vi "COD内部交互全局.vi"() -> ()   [LabVIEW 2016, in "斯坦道CODMn.lvlib"]
panel:
  in  "PID参数":cluster{"P":dbl, "I":dbl, "D":dbl}
  out "F0-F5":u16[](array[numeric])
  in  "更换泵管":bool
  out "采水泵参数":i32[](array[numeric])
  in  "泵校准参数":T1
  in  "保存参数":dbl[](array[numeric])
  in  "选项卡控件":enum32{"滴定曲线", "温度曲线"}(tab)
  out "ORP滴定曲线":u16[](graph)
  out "滴定数-ORP值":u16[](array[numeric]) caption="数组"
  out "波形时间":timestamp
  out "时间温度曲线":u16[](graph)
  out "时间-温度":u16[](array[numeric]) caption="数组"
  out "温度波形时间":timestamp
  out "第一次测试时间":timestamp
  in  "基本量程存储数据用":enum16{"L", "H", "AUTO"}(ring)
  out "报警点位":bool[](array[boolean])
  out "启用的浓度数组":dbl[](array[numeric])
  out "ORP显示":dbl
  out "实时温度":dbl
  out "高锰酸钾":dbl
  out "断电排液标记":bool
  out "报警簇":T2
  out "高锰酸钾报警":bool
  out "待机":bool
  in  "量程切换次数":u8
  out "测量模式数字":i32
  out "切换量程连续测两次":bool
  out "配置文件ini":string="data\\Set.ini"
  out "序列号:":string
  out "读取浮台参数显示":bool
  out "读取浮台参数":u16[](array[numeric])
  out "读取公式":u16[](array[numeric])
  out "读取参数":u16[](array[numeric])
  out "数据存储":u16[](array[numeric])
  out "温度":bool[](array[boolean])
  out "M输出点":bool[](array[boolean])
  out "ORP、时间":u16[](array[numeric])
  out "测量状态":u16[](array[numeric])
  out "读取公式显示":bool
  out "读取参数显示":bool
  out "读取写入data":bool
  in  "基本量程实时读取":enum16{"L", "H", "AUTO"}(ring)
  out "温度存储数据用":dbl
  out "故障标记":bool
  out "数据存储时间戳":timestamp format="%<%Y/%m/%d %H:%M:%S>T"
  out "通讯状态":bool
  out "data":T3
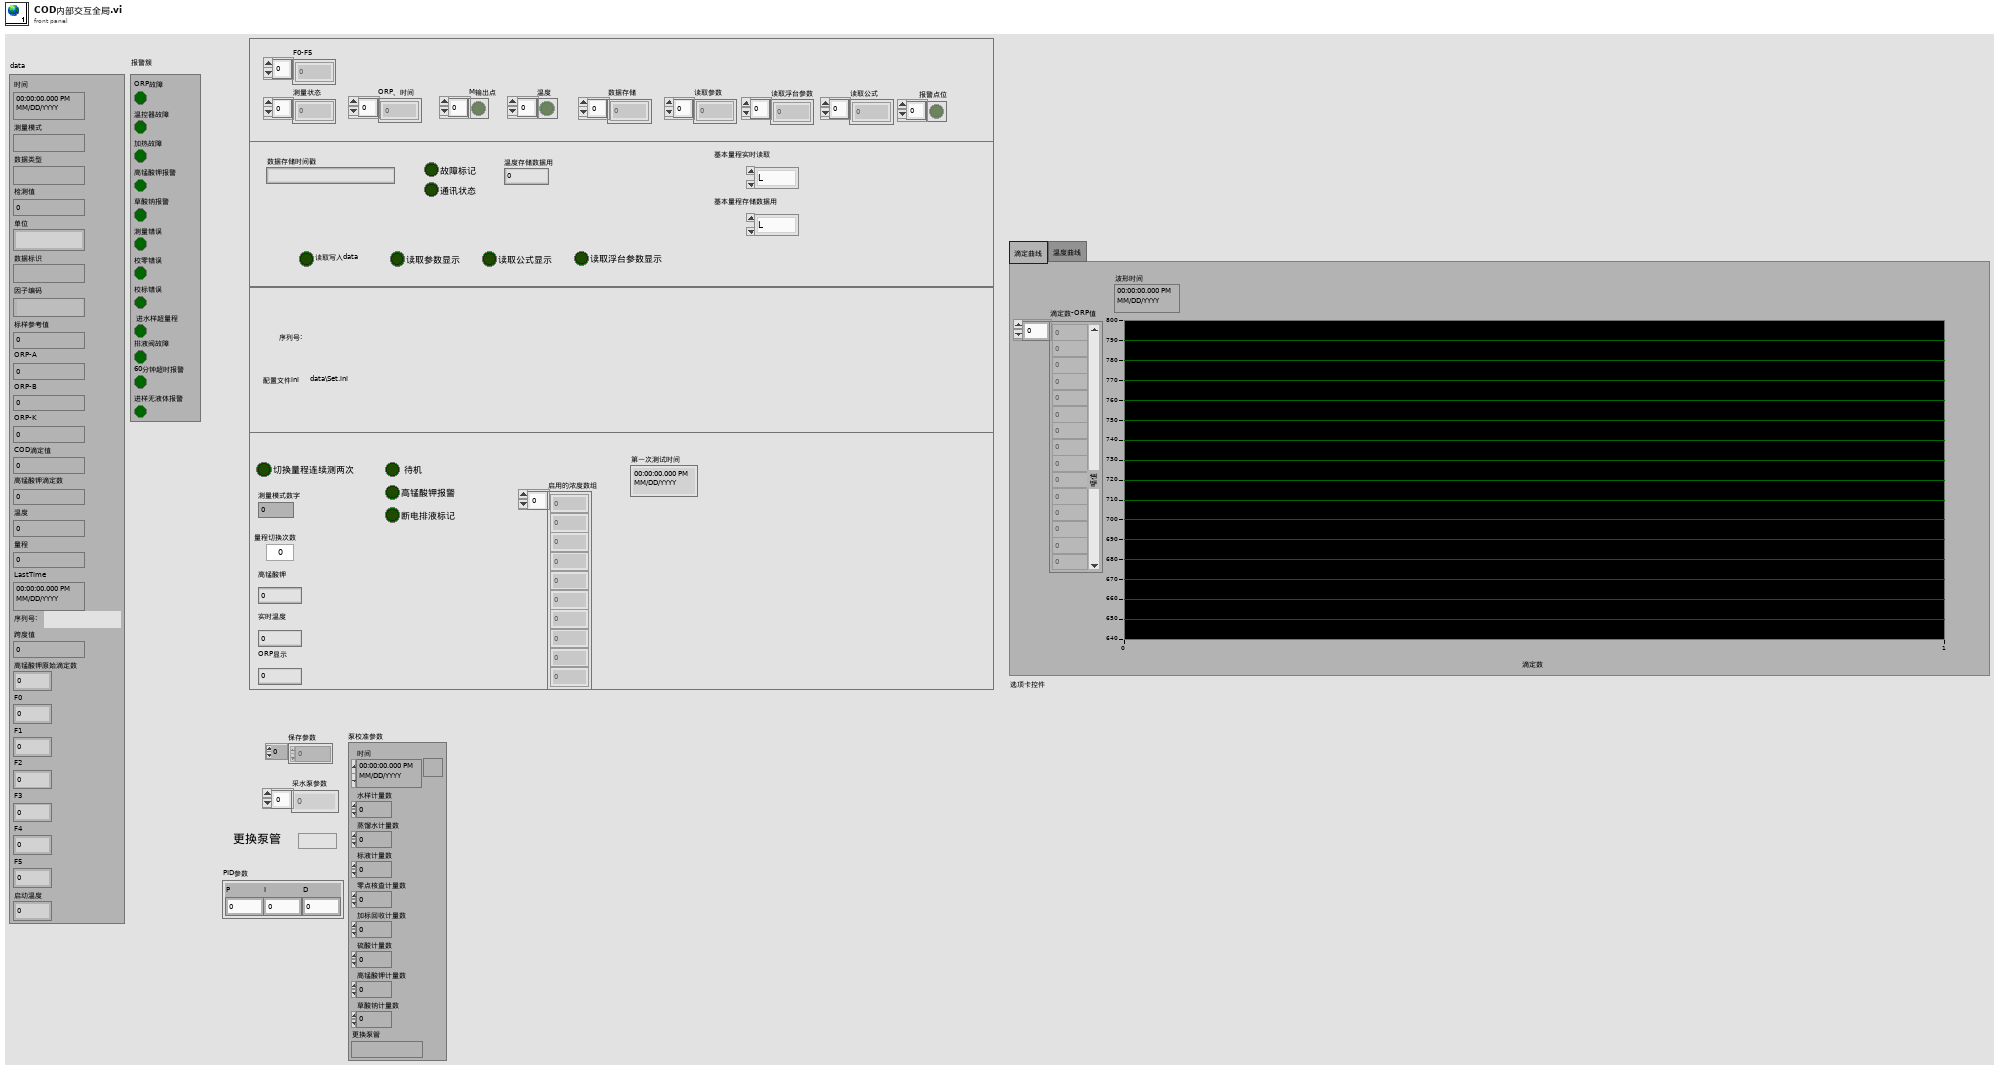
[diagram p1: front panel]
types:
  T1 = cluster{"时间":timestamp, "水样计量数":u16, "蒸馏水计量数":u16, "标液计量数":u16, "零点核查计量数":u16, "加标回收计量数":u16, "硫酸计量数":u16, "高锰酸钾计量数":u16, "草酸钠计量数":u16, "更换泵管":string}
  T2 = cluster{"ORP故障":bool, "温控器故障":bool, "加热故障":bool, "高锰酸钾报警":bool, "草酸钠报警":bool, "测量错误":bool, "校零错误":bool, "校标错误":bool, " 进水样超量程":bool, "排液阀故障":bool, "60分钟超时报警":bool, "进样无液体报警":bool}
  T3 = cluster{"时间":timestamp, "测量模式":string, "数据类型":string, "检测值":sgl, "单位":string, "数据标识":string, "因子编码":string, "标样参考值":sgl, "ORP-A":sgl, "ORP-B":sgl, "ORP-K":sgl, "COD滴定值":sgl, "高锰酸钾滴定数":sgl, "温度":sgl, "量程":sgl, "LastTime":timestamp, "序列号:":string, "跨度值":sgl, "高锰酸钾原始滴定数":sgl, "F0":sgl, "F1":sgl, "F2":sgl, "F3":sgl, "F4":sgl, "F5":sgl, "启动温度":sgl}
diagram:
